vi "FunArea.vi"(9 "Settings":T2 {"mag/phase" items=["FRF", "rad phase unwrapped", "deg phase unwrapped", "rad phase wrapped", "deg phase wrapped", "White Plots", "MJ Map", "Real and Imaginary"]; "Bands" items=["No Bands", "", "Test2", "test3", "Test"]; "Smoothing" items=["No smoothing"=0, "1/4 semitone"=25, "1/2 semitone"=50, "1 semitone"=100, "2 semitones"=200, "Woodhouse"=19]; "View Type" items=["As measured", "Normalize", "Separate", "Complex Average", "Real Average", "Standard Deviation"]}, 11 "Old Files":T3[](array[typedef])) -> ()   [LabVIEW 2022 SP3]
uses:
  Curtin1_Label.ctl
  GraphType.ctl
  Mic/Mic_Global.vi
panel:
  in  "compare instruments":bool
  in  "convolve":bool
  in  "Bridge":bool
  in  "Sorting":bool
  in  "2D plots":bool
  in  "WAV - MJ":bool
  in  "CSV":bool
  in  "White":bool
  in  "Tom King":bool
  in  "Woodhouse":bool
  in  "UFF":bool
  in  "Waveforms":bool
  in  "Marty":bool
  in  "Convert":bool
  in  "Colin":bool
  in  "live":bool
  in  "play":bool
  in  "Math":bool
  in  "Check Prefs":bool
  # "this is a place where we will add fun stuff - like hearing your waveform files, convolving your FRF with an input, viewing raw data, a real-time spectrograph etc"
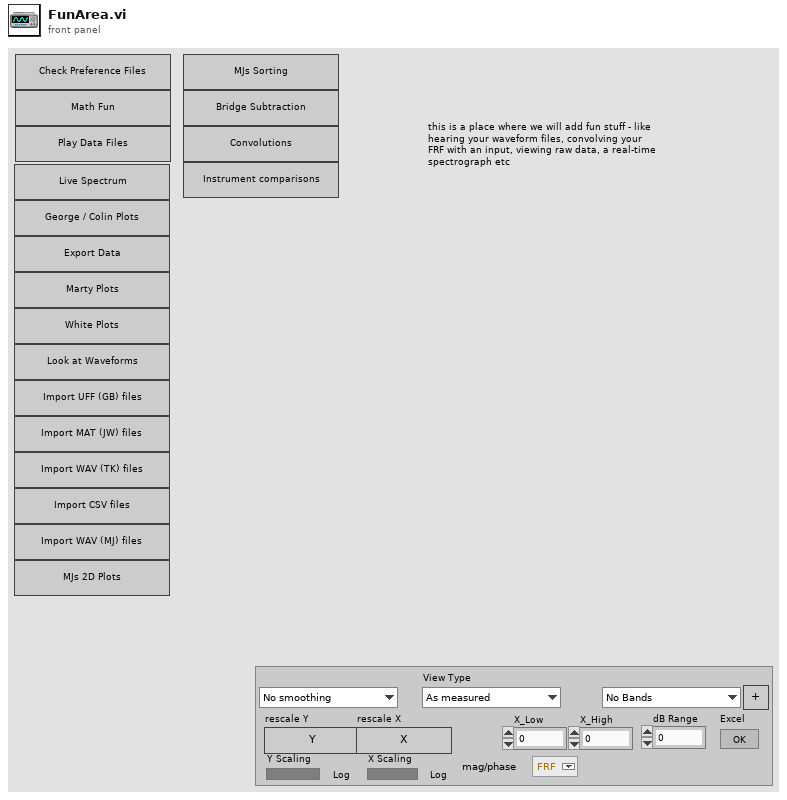
[diagram p1: front panel]
types:
  T1 = typedef "GraphType.ctl" = u16
  T2 = cluster{"View Type":u16, "Smoothing":u16, "Bands":u16, "New Band":bool, "rescale Y":bool, "rescale X":bool, "X_Low":dbl, "X_High":dbl, "dB Range":dbl, "Excel":bool, "Y Scaling":bool, "X Scaling":bool, "mag/phase":T1}
  T3 = typedef "Curtin1_Label.ctl" = cluster{"Show?":bool, "Name":string, "Color":u32, "Path":path, "Show Notes":bool}
  T4 = typedef "PreferencesControl.ctl" = cluster{"Name of test":string, "Date":timestamp, "Location":string, "Template":string, "Soundcard":string, "resolution":u16, "Sampling rate":u16, "Ch1 Gain ":dbl, "Ch2 Gain":dbl, "Sample time (s)":dbl, "Pre-trigger (s)":dbl, "Hammer Threshold":dbl, "Positions":i16, "Taps/Position":i16, "Set Names":string, "Freq resolution":dbl, "Hammer cutoff":dbl, "Mic cutoff":dbl, "Double bounce ":dbl, "Hammer Cal":dbl, "dB Offset":dbl, "Accel Cal":dbl, "Vibrometer Cal":dbl, "Mic Cal":dbl, "Output":u16, "Voltage Cal":dbl, "Vibrometer Port":refnum<visa-resource-name>, "Range":u16, "High Pass":u16, "Bandwidth":u16, "X Range":cluster{"Minimum":dbl, "Maximum":dbl, "Increment":dbl, "Minor Increment":dbl, "Start":dbl}[], "Y Range":cluster{"Minimum":dbl, "Maximum":dbl, "Increment":dbl, "Minor Increment":dbl, "Start":dbl}[], "dB Spread":dbl, "Trigger":u16, "Ch_1":u8, "Ch_2":u8, "flip?":bool, "60Hz":bool, "Time offset":dbl, "Piezo Cal":dbl, "Default Notes":string}
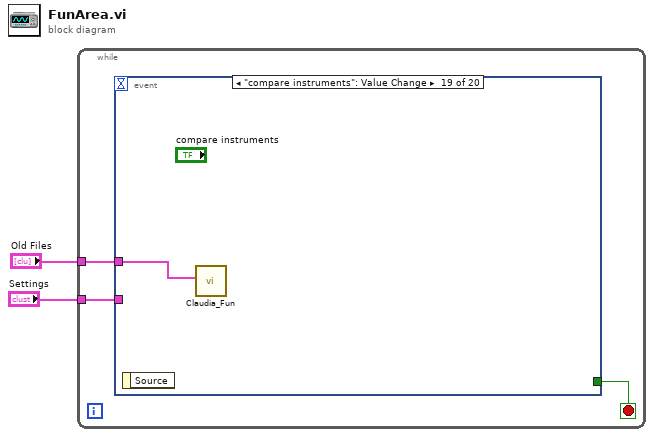
[diagram p0: block diagram]
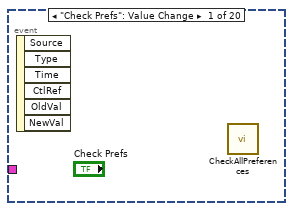
[diagram p2: hidden frame]
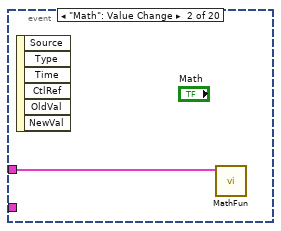
[diagram p3: hidden frame]
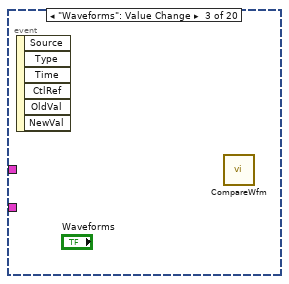
[diagram p4: hidden frame]
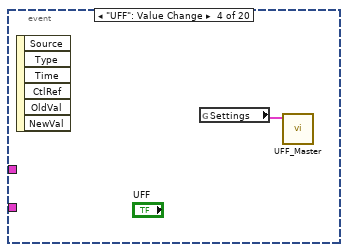
[diagram p5: hidden frame]
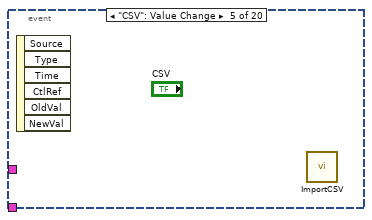
[diagram p6: hidden frame]
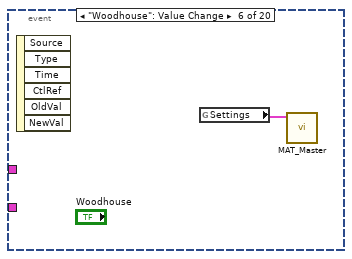
[diagram p7: hidden frame]
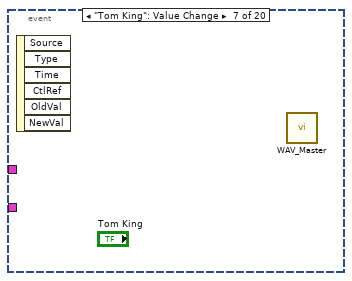
[diagram p8: hidden frame]
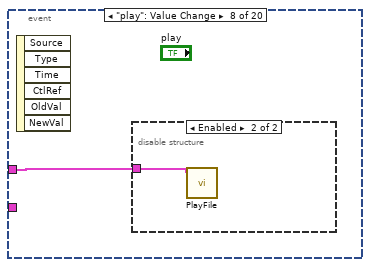
[diagram p9: hidden frame]
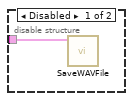
[diagram p10: hidden frame]
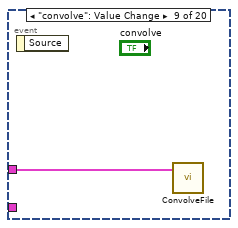
[diagram p11: hidden frame]
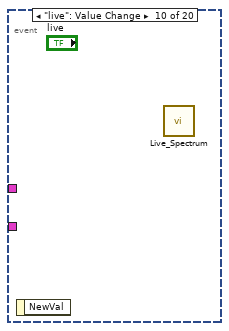
[diagram p12: hidden frame]
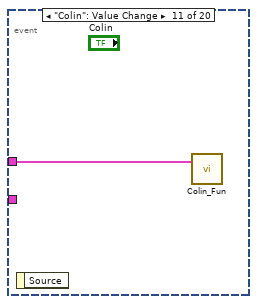
[diagram p13: hidden frame]
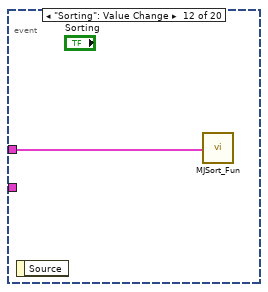
[diagram p14: hidden frame]
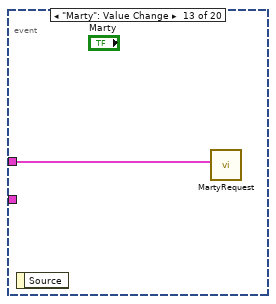
[diagram p15: hidden frame]
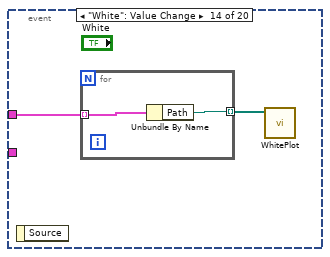
[diagram p16: hidden frame]
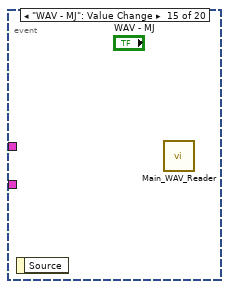
[diagram p17: hidden frame]
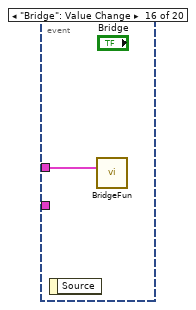
[diagram p18: hidden frame]
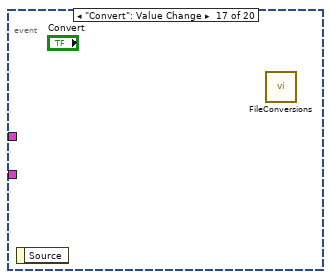
[diagram p19: hidden frame]
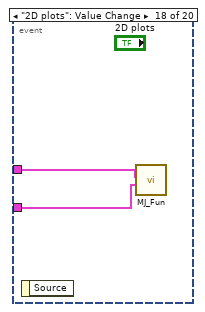
[diagram p20: hidden frame]
diagram:
  n1 = while {
    tunnel: "Old Files" -> [w4]
    tunnel: "Settings" -> [w3]
    stop <- w5 stop-if-true
    n2 = event shown="[18] \"compare instruments\": Value Change" {
      selector: _ -> [_ _ _ _ _ _ _ _ _ _ _ _ _ _ _ _ _ _ _ _]
      dyn-events: _ -> [_ _ _ _ _ _ _ _ _ _ _ _ _ _ _ _ _ _ _ _]
      timeout: _ -> [_ _ _ _ _ _ _ _ _ _ _ _ _ _ _ _ _ _ _ _]
      tunnel: [_ _ _ _ _ _ _ _ _ _ _ _ _ _ _ _ _ _ _ TRUE] -> w5
      tunnel: w4 -> [_ w6 _ _ _ _ _ w9 w12 _ w13 w14 w15 w17 _ w20 _ w22 w23 _]
      tunnel: w3 -> [_ _ _ _ _ _ _ _ _ _ _ _ _ _ _ _ _ w21 _ _]
      event "Check Prefs": Value Change {
        n3 = event-data() -> ()  [unwired: 1 in, 6 out]
        n4 = call "CheckAllPreferences.vi"() -> ()  [unwired: 12 in]
      }
      event "Math": Value Change {
        n5 = event-data() -> ()  [unwired: 1 in, 6 out]
        n6 = call "MathFun.vi"("Old Files"=w6) -> ()  [unwired: 11 in]
      }
      event "Waveforms": Value Change {
        n7 = event-data() -> ()  [unwired: 1 in, 6 out]
        n8 = call "CompareWfm.vi"() -> ()  [unwired: 12 in]
      }
      event "UFF": Value Change {
        n9 = event-data() -> ()  [unwired: 1 in, 6 out]
        n10 = global read "Mic_Global.vi" "Settings"() -> (w7:T4)
        n11 = call "UFF_Master.vi"("Settings in"=w7) -> ()  [unwired: 11 in]
      }
      event "CSV": Value Change {
        n12 = event-data() -> ()  [unwired: 1 in, 6 out]
        n13 = call "ImportCSV.vi"() -> ()  [unwired: 12 in]
      }
      event "Woodhouse": Value Change {
        n14 = event-data() -> ()  [unwired: 1 in, 6 out]
        n15 = global read "Mic_Global.vi" "Settings"() -> (w8:T4)
        n16 = call "MAT_Master.vi"("Settings in"=w8) -> ()  [unwired: 11 in]
      }
      event "Tom King": Value Change {
        n17 = event-data() -> ()  [unwired: 1 in, 6 out]
        n18 = call "WAV_Master.vi"() -> ()  [unwired: 12 in]
      }
      event "play": Value Change {
        n19 = event-data() -> ()  [unwired: 1 in, 6 out]
        n20 = disable-structure shown="Enabled" {
          disable-tunnel: w9 -> [w10 w11]
          frame Disabled {
            n21 = call "SaveWAVFile.vi"("Old Files"=w10) -> ()  [unwired: 11 in]
          }
          frame Enabled {
            n22 = call "PlayFile.vi"("Old Files"=w11) -> ()  [unwired: 11 in]
          }
        }
      }
      event "convolve": Value Change {
        n23 = event-data() -> ()  [unwired: 1 in, 1 out]
        n24 = call "ConvolveFile.vi"("Old Files"=w12) -> ()  [unwired: 11 in]
      }
      event "live": Value Change {
        n25 = event-data() -> ()  [unwired: 1 in, 1 out]
        n26 = call "Live_Spectrum.vi"() -> ()  [unwired: 12 in]
      }
      event "Colin": Value Change {
        n27 = event-data() -> ()  [unwired: 1 in, 1 out]
        n28 = call "Colin_Fun.vi"("Old Files"=w13) -> ()  [unwired: 11 in]
      }
      event "Sorting": Value Change {
        n29 = event-data() -> ()  [unwired: 1 in, 1 out]
        n30 = call "MJSort_Fun.vi"("Old Files"=w14) -> ()  [unwired: 11 in]
      }
      event "Marty": Value Change {
        n31 = event-data() -> ()  [unwired: 1 in, 1 out]
        n32 = call "MartyRequest.vi"("Old Files"=w15) -> ()  [unwired: 11 in]
      }
      event "White": Value Change {
        n33 = event-data() -> ()  [unwired: 1 in, 1 out]
        n34 = for {
          tunnel: w17 -> [w19] mode=indexing
          tunnel: [w18] -> w16 mode=indexing
          n35 = Unbundle By Name(w19) -> ("Path"=w18:path)
        }
        n36 = call "WhitePlot.vi"("Paths"=w16) -> ()  [unwired: 11 in]
      }
      event "WAV - MJ": Value Change {
        n37 = event-data() -> ()  [unwired: 1 in, 1 out]
        n38 = call "Main_WAV_Reader.vi"() -> ()  [unwired: 12 in]
      }
      event "Bridge": Value Change {
        n39 = event-data() -> ()  [unwired: 1 in, 1 out]
        n40 = call "BridgeFun.vi"("Files"=w20) -> ()  [unwired: 11 in]
      }
      event "Convert": Value Change {
        n41 = event-data() -> ()  [unwired: 1 in, 1 out]
        n42 = call "FileConversions.vi"() -> ()  [unwired: 12 in]
      }
      event "2D plots": Value Change {
        n43 = event-data() -> ()  [unwired: 1 in, 1 out]
        n44 = call "MJ_Fun.vi"("Views"=w21, "Old Files"=w22) -> ()  [unwired: 10 in]
      }
      event "compare instruments": Value Change {
        n45 = event-data() -> ()  [unwired: 1 in, 1 out]
        n46 = call "Claudia_Fun.vi"("Files"=w23) -> ()  [unwired: 11 in]
      }
      event Panel Close {
        n47 = event-data() -> ()  [unwired: 1 in, 4 out]
      }
    }
  }
